vi "MPExxx_set_trigger.vi"(0 "VISA session":refnum<visa-resource-name>, 1 "Set Trigger Voltage":dbl format="%.2f", 2 "Set Trigger Current":dbl format="%.2f", 3 "error in (no error)":errorcluster, 4 "Initiate Continuous":bool) -> (5 "dup VISA session":refnum<visa-resource-name>, 6 "error out":errorcluster)   [LabVIEW 2012]
doc: "This VI form sets the triggering mode for the power supply. It sets the trigger levels and the initiate continuous discrete."
panel:
  # "MAGNA-POWER"
  # "Electronics"
  # "ON"
  # "OFF"
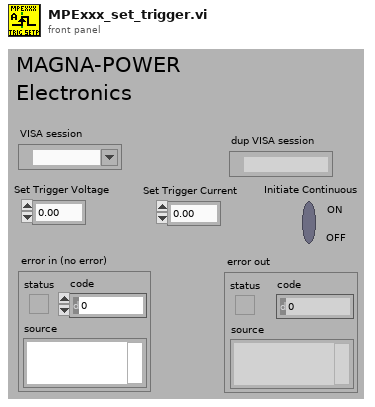
[diagram p1: front panel]
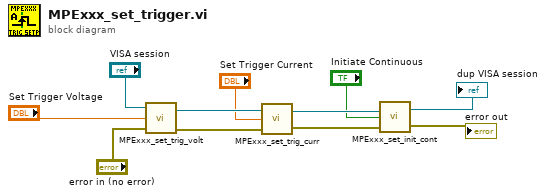
[diagram p0: block diagram]
diagram:
  n1 = call "MPExxx_set_trig_volt.vi"("error in (no error)"="error in (no error)", "Set Trigger Voltage"="Set Trigger Voltage", "VISA session"="VISA session") -> ("error out"=w8:errorcluster, "dup VISA session"=w11:refnum<visa-resource-name>)
  n2 = call "MPExxx_set_trig_curr.vi"("error in (no error)"=w8, "Set Trigger Current"="Set Trigger Current", "VISA session"=w11) -> ("error out"=w9:errorcluster, "dup VISA session"=w10:refnum<visa-resource-name>)
  n3 = call "MPExxx_set_init_cont.vi"("error in (no error)"=w9, "Initiate Continuous"="Initiate Continuous", "VISA session"=w10) -> ("error out"=→"error out":errorcluster, "dup VISA session"=→"dup VISA session":refnum<visa-resource-name>)
